vi "PlotMetaAllCH.vi"(0 "object in":refnum<class "AD2_MSO_SDK.lvclass">, 5 "error in (no error)":errorcluster) -> (14 "object out":refnum<class "AD2_MSO_SDK.lvclass">, 15 "Waveform Graph 2":waveform(dbl)[](graph)=[{"t0"=timestamp(0 s since 1904-01-01), "dt"=1e-06, "Y"=array[8192 elements]}, {"t0"=timestamp(0 s since 1904-01-01), "dt"=1e-06, "Y"=array[8192 elements]}], 16 "MetaData":T1 {"Ch 2"."detected frequency" format="%.2p"; "Ch 2"."detected amplitude" format="%.2p"; "Ch 2"."detected phase (deg)" format="%.2p"; "Ch 1"."detected frequency" format="%.2p"; "Ch 1"."detected amplitude" format="%.2p"; "Ch 1"."detected phase (deg)" format="%.2p"}, 19 "error out":errorcluster)   [LabVIEW 2019, in "AD2_MSO_SDK.lvclass"]
uses:
  AD2_MSO_SDK.lvclass
  <vilib>/measure/matone.llb/Extract Single Tone Information 1 Chan.vi
  <vilib>/measure/NI_MAPro.lvlib
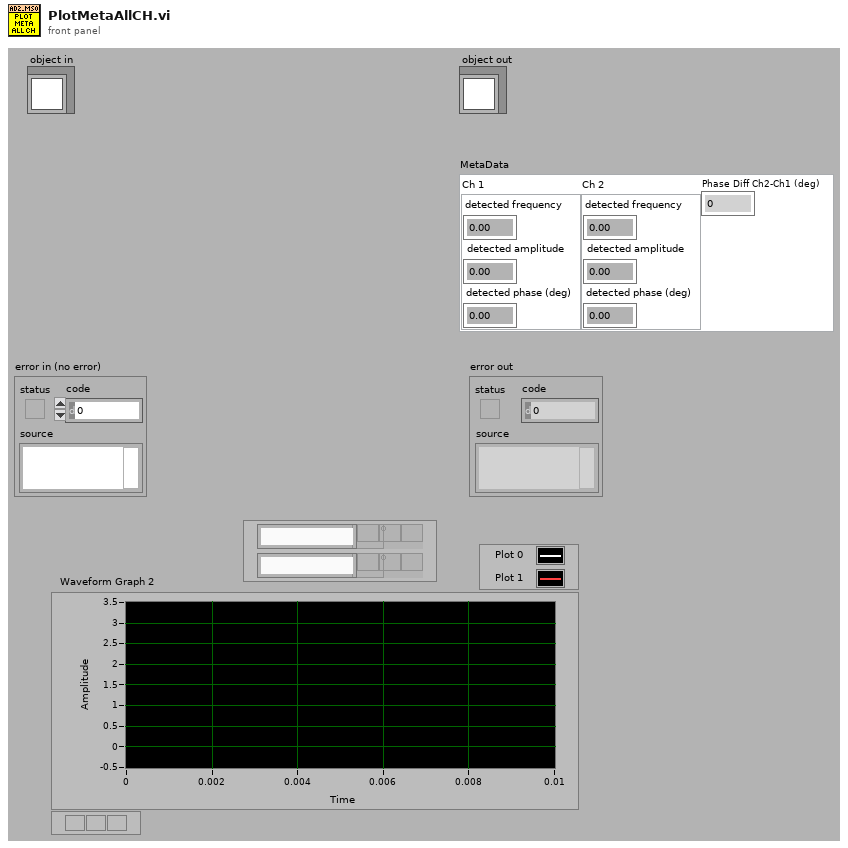
[diagram p1: front panel]
types:
  T1 = cluster{"Ch 1":cluster{"detected frequency":dbl, "detected amplitude":dbl, "detected phase (deg)":dbl}, "Ch 2":cluster{"detected frequency":dbl, "detected amplitude":dbl, "detected phase (deg)":dbl}, "Phase Diff Ch2-Ch1 (deg)":dbl}
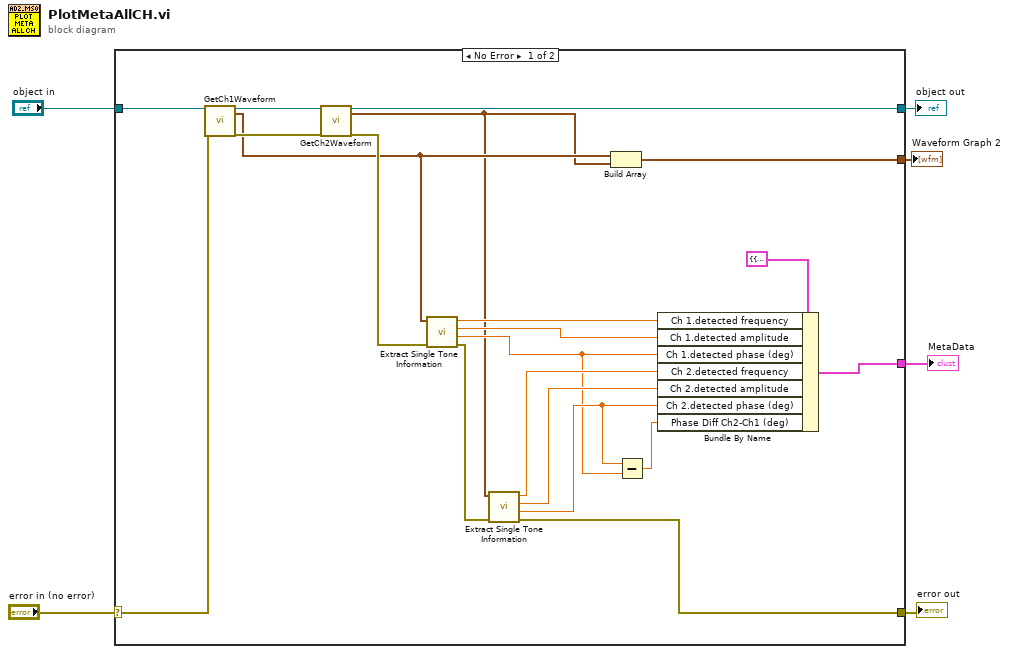
[diagram p0: block diagram]
diagram:
  n1 = case shown="No Error" "error in (no error)" {
    selector: "error in (no error)" -> [w21 w28]
    tunnel: [w20 w28] -> w5
    tunnel: [w24 w27] -> w3
    tunnel: "object in" -> [w23 w27]
    tunnel: [w26 _] -> w2
    tunnel: [w11 _] -> w1
    frame No Error {
      n2 = call-dynamic "GetCh1Waveform.vi"("object in"=w23, "error in (no error)"=w21) -> ("object out"=w25:refnum<class "AD2_MSO_SDK.lvclass">, "Ch1 waveform"=w8:waveform(dbl), "error out"=w22:errorcluster)  [unwired: 15 in]
      n3 = call-dynamic "GetCh2Waveform.vi"("object in"=w25, "error in (no error)"=w22) -> ("object out"=w24:refnum<class "AD2_MSO_SDK.lvclass">, "Ch2 waveform"=w7:waveform(dbl), "error out"=w19:errorcluster)  [unwired: 15 in]
      n4 = call-poly <vilib>:"Extract Single Tone Information.vi"("error in (no error)"=w19, "time signal in"=w8) -> ("error out"=w18:errorcluster, "detected phase (deg)"=w12:dbl, "detected amplitude"=w16:dbl, "detected frequency"=w17:dbl)  [unwired: 4 in, 2 out]
      n5 = call-poly <vilib>:"Extract Single Tone Information.vi"("error in (no error)"=w18, "time signal in"=w7) -> ("error out"=w20:errorcluster, "detected phase (deg)"=w13:dbl, "detected amplitude"=w14:dbl, "detected frequency"=w15:dbl)  [unwired: 4 in, 2 out]
      n6 = Build Array(w8, w7) -> (w26:waveform(dbl)[])
      n7 = Subtract(x=w13, y=w12) -> (x-y=w9:dbl)
      n8 = Bundle By Name(cluster=T1 {"Ch 1"={"detected frequency"=0.0, "detected amplitude"=0.0, "detected phase (deg)"=0.0}, "Ch 2"={"detected frequency"=0.0, "detected amplitude"=0.0, "detected phase (deg)"=0.0}, "Phase Diff Ch2-Ch1 (deg)"=0.0} ("MetaData"), "Ch 1.detected frequency"=w17, "Ch 1.detected amplitude"=w16, "Ch 1.detected phase (deg)"=w12, "Ch 2.detected frequency"=w15, "Ch 2.detected amplitude"=w14, "Ch 2.detected phase (deg)"=w13, "Phase Diff Ch2-Ch1 (deg)"=w9) -> (w11:T1)
    }
    frame Error {
    }
  }
  "error out" <- w5
  "object out" <- w3
  "Waveform Graph 2" <- w2
  "MetaData" <- w1
